vi "getLabels.vi"(7 "LabVIEW Web Service Request":refnum<class "Web Request.lvclass">) -> ()   [LabVIEW 2016]
uses:
  <vilib>/wsapi/Web Request.lvclass
  Typedef/MAC & Labels.ctl
  <vilib>/Utility/file.llb/Read Delimited Spreadsheet (string).vi
  <userlib>/_OpenG.lib/array/array.llb/Remove Duplicates from 1D Array (String)__ogtk.vi
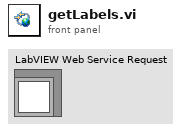
[diagram p1: front panel]
types:
  T1 = typedef "MAC & Labels.ctl" = cluster{"MAC list":string[], "Label list":string[]}
  T2 = enum16{"open", "replace", "create", "open or create", "replace or create", "replace or create with confirmation"}
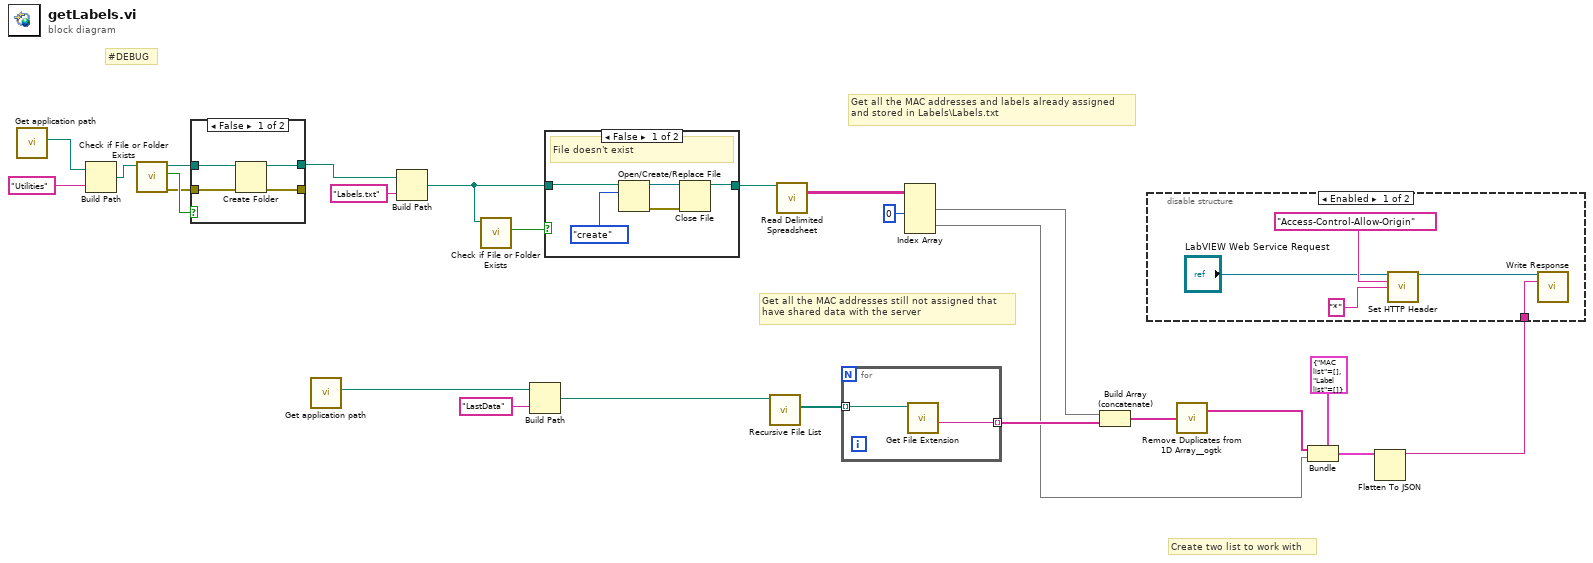
[diagram p0: block diagram]
diagram:
  # "#DEBUG"
  # "Create two list to work with"
  # "Get all the MAC addresses still not assigned that\nhave shared data with the server"
  # "Get all the MAC addresses and labels already assigned\nand stored in Labels\\Labels.txt"
  n1 = call "Get application path.vi"() -> ("Application path"=w2:path)  [unwired: 11 in]
  n2 = Build Path(base path=w2, name or relative path="Utilities") -> (appended path=w4:path)
  n3 = call <vilib>:"Check if File or Folder Exists.vi"("path"=w4) -> ("error out"=w8:errorcluster, "file or folder exists?"=w9:bool, "dup path"=w7:path)  [unwired: 8 in]
  n4 = case shown="False" w9 {
    tunnel: w8 -> [w29 w30]
    tunnel: w7 -> [w28 w31]
    tunnel: [w27 w31] -> w6
    tunnel: [w26 w30] -> _
    frame False {
      n5 = Create Folder(path (use dialog)=w28, error in=w29) -> (created path=w27:path, error out=w26:errorcluster)  [unwired: 1 in, 1 out]
    }
    frame True {
    }
  }
  n6 = call "Get application path.vi"() -> ("Application path"=w1:path)  [unwired: 11 in]
  n7 = Build Path(base path=w6, name or relative path="Labels.txt") -> (appended path=w11:path)
  n8 = call <vilib>:"Check if File or Folder Exists.vi"("path"=w11) -> ("file or folder exists?"=w12:bool)  [unwired: 8 in, 2 out]
  n9 = Build Path(base path=w1, name or relative path="LastData") -> (appended path=w25:path)
  n10 = case shown="False" w12 {
    tunnel: [w33 w37] -> w13
    tunnel: w11 -> [w32 w37]
    frame False {
      # "File doesn't exist"
      n11 = Open/Create/Replace File(file path (use dialog)=w32, operation (0:open)=T2."create") -> (refnum out=w34:refnum<file>, error out=w35:errorcluster)  [unwired: 4 in, 1 out]
      n12 = Close File(refnum=w34, error in=w35) -> (path=w33:path)  [unwired: 1 out]
    }
    frame True {
      # "File exist"
    }
  }
  n13 = call <vilib>:"Recursive File List.vi"("Folder Path"=w25) -> ("All Files in Dir"=w24:path[])  [unwired: 6 in, 4 out]
  n14 = call-poly <vilib>:"Read Delimited Spreadsheet.vi"("file path (dialog if empty)"=w13) -> ("all rows"=w22:string[][])  [unwired: 9 in, 5 out]
  n15 = for {
    tunnel: w24 -> [w39] mode=indexing
    tunnel: [w38] -> w19 mode=indexing
    n16 = call <vilib>:"Get File Extension.vi"("file"=w39) -> ("filename without extension"=w38:string)  [unwired: 6 in, 4 out]
  }
  n17 = Index Array(array=w22, index (col) #1=0 ("disabled index (col)")) -> (element #1=w20:string[], element #2=w16:string[])  [unwired: 3 in]
  n18 = Build Array (concatenate)(w20, w19) -> (w18:string[])
  n19 = call-poly <userlib>:"Remove Duplicates from 1D Array__ogtk.vi"("Input Array"=w18) -> ("Output Array"=w17:string[])  [unwired: 1 out]
  n20 = Bundle(cluster=T1 {"MAC list"=[], "Label list"=[]}, "MAC list"=w17, "Label list"=w16) -> (w15:T1)
  n21 = Flatten To JSON(anything=w15) -> (JSON string=w23:string)  [unwired: 2 in, 1 out]
  n22 = disable-structure shown="Enabled" {
    disable-tunnel: w23 -> [w44 _]
    frame Enabled {
      n23 = call <vilib>:"Set HTTP Header.vi"("LabVIEW Web Service Request"="LabVIEW Web Service Request", "header"="Access-Control-Allow-Origin", "header value"="*") -> ("LabVIEW Web Service Request out"=w40:refnum<class "Web Request.lvclass">)  [unwired: 11 in, 1 out]
      n24 = call <vilib>:"Write Response.vi"("LabVIEW Web Service Request"=w40, "response string"=w44) -> ()  [unwired: 12 in, 2 out]
    }
    frame Disabled {
    }
  }
